vi "to_array.vi"(8 "error in":errorcluster, 11 "labels in":refnum<class "labels.lvclass">) -> (0 "error out":errorcluster, 2 "Labels Array":string[](array[string]), 3 "labels out":refnum<class "labels.lvclass">)   [LabVIEW 2020, in "nominal types.lvlib" / "labels.lvclass"]
uses:
  labels.lvclass
  labels.lvclass/labels.ctl
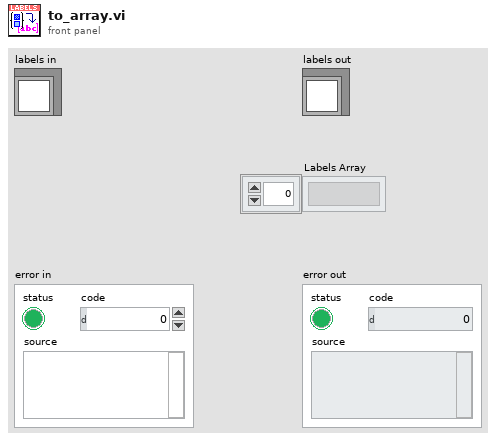
[diagram p1: front panel]
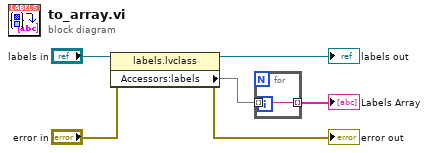
[diagram p0: block diagram]
diagram:
  n1 = property class="labels.lvclass"(reference="labels in", error in="error in") -> (reference out=→"labels out":refnum<class "labels.lvclass">, error out=→"error out":errorcluster, "Accessors:labels"=w5:set{string})
  n2 = for {
    tunnel: w5 -> [w7] mode=indexing
    tunnel: [w7] -> w4 mode=indexing
  }
  "Labels Array" <- w4
